vi "RconLookup.vi"(11 "iteration":i32 format="%02x") -> (3 "LookUp-Out":u8[](array[numeric]) format="%02x")   [LabVIEW 2011, in "i3-external-encryption.lvlib"]
doc: "Performs the R-con lookup for AES algorithm.\nThe output is a U32, with the first byte the Rcon-value, the rest is 0, to use in the XOR function.\n\n(c) Ton Plomp, 2011\nTHIS SOFTWARE IS PROVIDED AS IS, AND ANY WARRANTY IS REJECTED"
uses:
  i3-external-encryption.lvlib
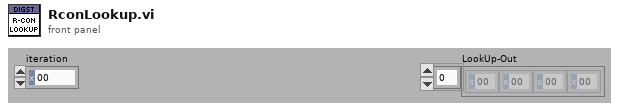
[diagram p1: front panel]
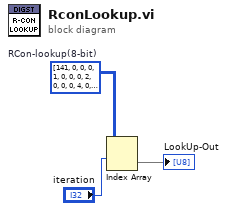
[diagram p0: block diagram]
diagram:
  w1 = u8[][] [[141, 0, 0, 0], [1, 0, 0, 0], [2, 0, 0, 0], [4, 0, 0, 0], [8, 0, 0, 0], [16, 0, 0, 0], [32, 0, 0, 0], [64, 0, 0, 0], [128, 0, 0, 0], [27, 0, 0, 0], [54, 0, 0, 0], [108, 0, 0, 0], [216, 0, 0, 0], [171, 0, 0, 0], [77, 0, 0, 0], [154, 0, 0, 0], [47, 0, 0, 0], [94, 0, 0, 0], [188, 0, 0, 0], [99, 0, 0, 0], [198, 0, 0, 0], [151, 0, 0, 0], [53, 0, 0, 0], [106, 0, 0, 0], [212, 0, 0, 0], [179, 0, 0, 0], [125, 0, 0, 0], [250, 0, 0, 0], [239, 0, 0, 0], [197, 0, 0, 0], [145, 0, 0, 0], [57, 0, 0, 0], [114, 0, 0, 0], [228, 0, 0, 0], [211, 0, 0, 0], [189, 0, 0, 0], [97, 0, 0, 0], [194, 0, 0, 0], [159, 0, 0, 0], [37, 0, 0, 0], [74, 0, 0, 0], [148, 0, 0, 0], [51, 0, 0, 0], [102, 0, 0, 0], [204, 0, 0, 0], [131, 0, 0, 0], [29, 0, 0, 0], [58, 0, 0, 0], [116, 0, 0, 0], [232, 0, 0, 0], [203, 0, 0, 0], [141, 0, 0, 0], [1, 0, 0, 0], [2, 0, 0, 0], [4, 0, 0, 0], [8, 0, 0, 0], [16, 0, 0, 0], [32, 0, 0, 0], [64, 0, 0, 0], [128, 0, 0, 0], [27, 0, 0, 0], [54, 0, 0, 0], [108, 0, 0, 0], [216, 0, 0, 0], [171, 0, 0, 0], [77, 0, 0, 0], [154, 0, 0, 0], [47, 0, 0, 0], [94, 0, 0, 0], [188, 0, 0, 0], [99, 0, 0, 0], [198, 0, 0, 0], [151, 0, 0, 0], [53, 0, 0, 0], [106, 0, 0, 0], [212, 0, 0, 0], [179, 0, 0, 0], [125, 0, 0, 0], [250, 0, 0, 0], [239, 0, 0, 0], [197, 0, 0, 0], [145, 0, 0, 0], [57, 0, 0, 0], [114, 0, 0, 0], [228, 0, 0, 0], [211, 0, 0, 0], [189, 0, 0, 0], [97, 0, 0, 0], [194, 0, 0, 0], [159, 0, 0, 0], [37, 0, 0, 0], [74, 0, 0, 0], [148, 0, 0, 0], [51, 0, 0, 0], [102, 0, 0, 0], [204, 0, 0, 0], [131, 0, 0, 0], [29, 0, 0, 0], [58, 0, 0, 0], [116, 0, 0, 0], [232, 0, 0, 0], [203, 0, 0, 0], [141, 0, 0, 0], [1, 0, 0, 0], [2, 0, 0, 0], [4, 0, 0, 0], [8, 0, 0, 0], [16, 0, 0, 0], [32, 0, 0, 0], [64, 0, 0, 0], [128, 0, 0, 0], [27, 0, 0, 0], [54, 0, 0, 0], [108, 0, 0, 0], [216, 0, 0, 0], [171, 0, 0, 0], [77, 0, 0, 0], [154, 0, 0, 0], [47, 0, 0, 0], [94, 0, 0, 0], [188, 0, 0, 0], [99, 0, 0, 0], [198, 0, 0, 0], [151, 0, 0, 0], [53, 0, 0, 0], [106, 0, 0, 0], [212, 0, 0, 0], [179, 0, 0, 0], [125, 0, 0, 0], [250, 0, 0, 0], [239, 0, 0, 0], [197, 0, 0, 0], [145, 0, 0, 0], [57, 0, 0, 0], [114, 0, 0, 0], [228, 0, 0, 0], [211, 0, 0, 0], [189, 0, 0, 0], [97, 0, 0, 0], [194, 0, 0, 0], [159, 0, 0, 0], [37, 0, 0, 0], [74, 0, 0, 0], [148, 0, 0, 0], [51, 0, 0, 0], [102, 0, 0, 0], [204, 0, 0, 0], [131, 0, 0, 0], [29, 0, 0, 0], [58, 0, 0, 0], [116, 0, 0, 0], [232, 0, 0, 0], [203, 0, 0, 0], [141, 0, 0, 0], [1, 0, 0, 0], [2, 0, 0, 0], [4, 0, 0, 0], [8, 0, 0, 0], [16, 0, 0, 0], [32, 0, 0, 0], [64, 0, 0, 0], [128, 0, 0, 0], [27, 0, 0, 0], [54, 0, 0, 0], [108, 0, 0, 0], [216, 0, 0, 0], [171, 0, 0, 0], [77, 0, 0, 0], [154, 0, 0, 0], [47, 0, 0, 0], [94, 0, 0, 0], [188, 0, 0, 0], [99, 0, 0, 0], [198, 0, 0, 0], [151, 0, 0, 0], [53, 0, 0, 0], [106, 0, 0, 0], [212, 0, 0, 0], [179, 0, 0, 0], [125, 0, 0, 0], [250, 0, 0, 0], [239, 0, 0, 0], [197, 0, 0, 0], [145, 0, 0, 0], [57, 0, 0, 0], [114, 0, 0, 0], [228, 0, 0, 0], [211, 0, 0, 0], [189, 0, 0, 0], [97, 0, 0, 0], [194, 0, 0, 0], [159, 0, 0, 0], [37, 0, 0, 0], [74, 0, 0, 0], [148, 0, 0, 0], [51, 0, 0, 0], [102, 0, 0, 0], [204, 0, 0, 0], [131, 0, 0, 0], [29, 0, 0, 0], [58, 0, 0, 0], [116, 0, 0, 0], [232, 0, 0, 0], [203, 0, 0, 0], [141, 0, 0, 0], [1, 0, 0, 0], [2, 0, 0, 0], [4, 0, 0, 0], [8, 0, 0, 0], [16, 0, 0, 0], [32, 0, 0, 0], [64, 0, 0, 0], [128, 0, 0, 0], [27, 0, 0, 0], [54, 0, 0, 0], [108, 0, 0, 0], [216, 0, 0, 0], [171, 0, 0, 0], [77, 0, 0, 0], [154, 0, 0, 0], [47, 0, 0, 0], [94, 0, 0, 0], [188, 0, 0, 0], [99, 0, 0, 0], [198, 0, 0, 0], [151, 0, 0, 0], [53, 0, 0, 0], [106, 0, 0, 0], [212, 0, 0, 0], [179, 0, 0, 0], [125, 0, 0, 0], [250, 0, 0, 0], [239, 0, 0, 0], [197, 0, 0, 0], [145, 0, 0, 0], [57, 0, 0, 0], [114, 0, 0, 0], [228, 0, 0, 0], [211, 0, 0, 0], [189, 0, 0, 0], [97, 0, 0, 0], [194, 0, 0, 0], [159, 0, 0, 0], [37, 0, 0, 0], [74, 0, 0, 0], [148, 0, 0, 0], [51, 0, 0, 0], [102, 0, 0, 0], [204, 0, 0, 0], [131, 0, 0, 0], [29, 0, 0, 0], [58, 0, 0, 0], [116, 0, 0, 0], [232, 0, 0, 0], [203, 0, 0, 0], [141, 0, 0, 0]]  # RCon-lookup(8-bit)
  n1 = Index Array(array=w1, index (row)="iteration") -> (element=→"LookUp-Out":u8[])  [unwired: 1 in]
